vi "Joystick.vi"(8 "error in":errorcluster, 10 "error in Linx":errorcluster, 11 "LINX Ref":T1) -> (0 "error out":errorcluster, 1 "Signals":cluster{"Switch":bool, "Ultrasonic":dbl}, 2 "Joystick":T7, 3 "Refnum out":refnum<k1>, 4 "error out Linx":errorcluster, 5 "LINX Ref":T1)   [LabVIEW 2013]
uses:
  <vilib>/LabVIEW Hacker/LINX/Private/Type Defs/LINX Ref.ctl
  <vilib>/LabVIEW Hacker/LINX/Private/Type Defs/Platform.ctl
  <vilib>/LabVIEW Hacker/LINX/Private/Type Defs/Interface.ctl
  <vilib>/LabVIEW Hacker/LINX/Private/Device/Type Defs/LINX Device Config.ctl
  <vilib>/LabVIEW Hacker/LINX/Private/Device/Type Defs/TCP Config.ctl
  <vilib>/LabVIEW Hacker/LINX/Private/Type Defs/Device Family.ctl
  <vilib>/Utility/inputDevices.llb/joystickAcquire.vi
  <vilib>/LabVIEW Hacker/LINX/Public/Peripherals/Analog/Analog Read 1 Chan.vi
  <vilib>/LabVIEW Hacker/LINX/Public/Peripherals/Digital/Digital Read 1 Chan.vi
  <vilib>/LabVIEW Hacker/LINX/LVH-LINX.lvlib
  <vilib>/LabVIEW Hacker/LINX/Private/Device/Device.lvlib
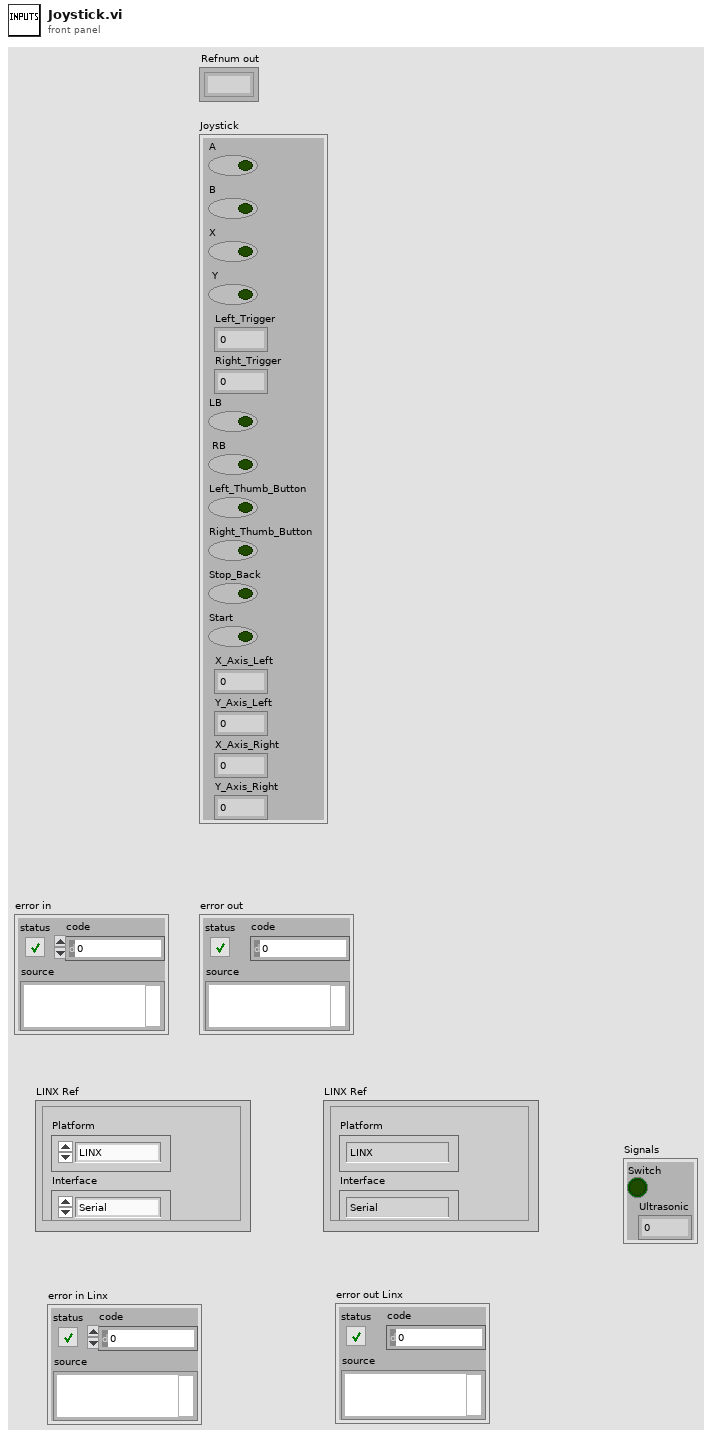
[diagram p1: front panel]
types:
  T1 = typedef "LVH-LINX.lvlib/LINX Ref.ctl" = cluster{"Platform":T2, "Interface":T3, "LINX Device Config":T4}
  T2 = typedef "LVH-LINX.lvlib/Platform.ctl" = enum16{"LINX", "myRIO"}
  T3 = typedef "LVH-LINX.lvlib/Interface.ctl" = enum16{"Serial", "TCP"}
  T4 = typedef "LVH-LINX.lvlib/Device.lvlib/LINX Device Config.ctl" = cluster{"Interface":T3, "COM Port":refnum<visa-resource-name>, "TCP Configuration":T5, "Device Family":T6, "Device ID":u8, "Device Name":string, "TCP Ref":refnum<k5>}
  T5 = typedef "LVH-LINX.lvlib/Device.lvlib/TCP Config.ctl" = cluster{"IP Address":string, "Port":u16}
  T6 = typedef "LVH-LINX.lvlib/Device Family.ctl" = enum8{"National Instruments", "Digilent", "Arduino"}
  T7 = cluster{"A":bool, "B":bool, "X":bool, " Y":bool, "Left_Trigger":dbl, "Right_Trigger ":dbl, "LB":bool, " RB":bool, "Left_Thumb_Button":bool, "Right_Thumb_Button":bool, "Stop_Back":bool, "Start":bool, "X_Axis_Left":dbl, "Y_Axis_Left":dbl, "X_Axis_Right":dbl, "Y_Axis_Right":dbl}
  T8 = cluster{"X axis":i32, "Y axis":i32, "Z axis":i32, "X axis rotation":i32, "Y axis rotation":i32, "Z axis rotation":i32, "U axis":i32, "V axis":i32}
  T9 = cluster{"button 1":bool, "button 2":bool, "button 3":bool, "button 4":bool, "button 5":bool, "button 6":bool, "button 7":bool, "button 8":bool, "button 9":bool, "button 10":bool, "button 11":bool, "button 12":bool, "button 13":bool, "button 14":bool, "button 15":bool, "button 16":bool, "button 17":bool, "button 18":bool, "button 19":bool, "button 20":bool, "button 21":bool, "button 22":bool, "button 23":bool, "button 24":bool, "button 25":bool, "button 26":bool, "button 27":bool, "button 28":bool, "button 29":bool, "button 30":bool, "button 31":bool, "button 32":bool}
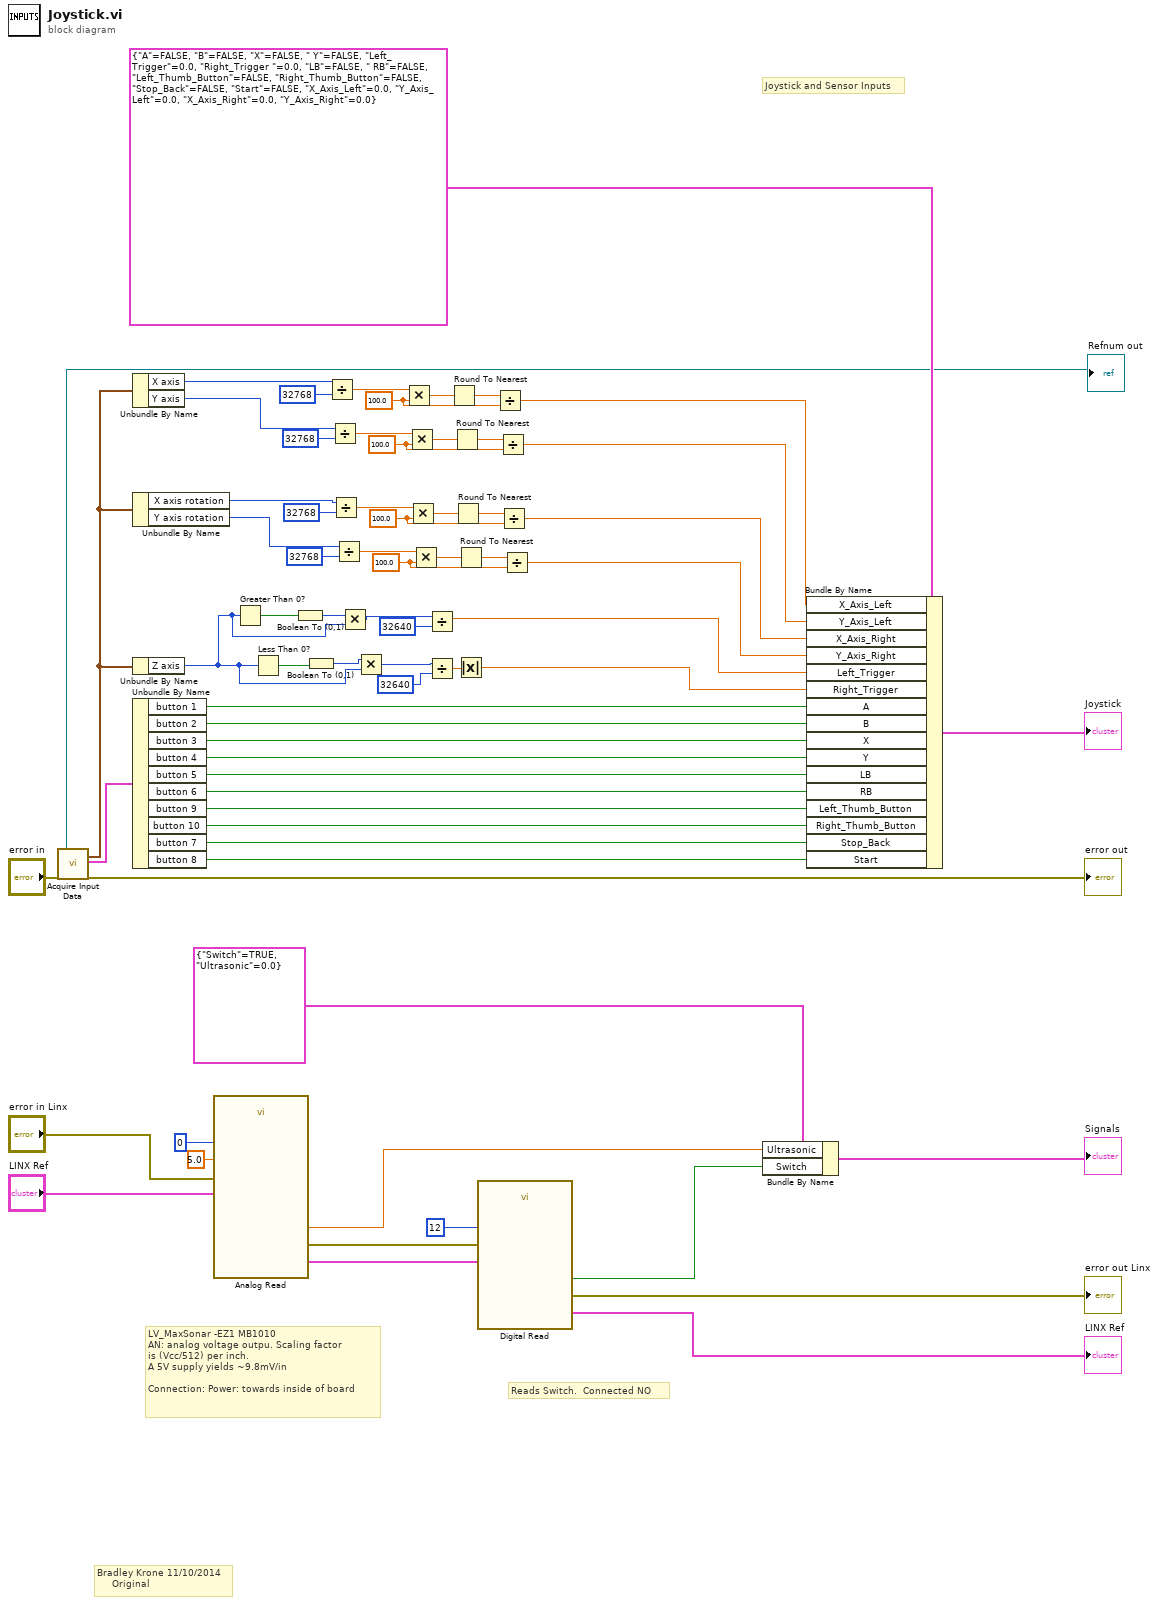
[diagram p0: block diagram]
diagram:
  w63 = 100.0 ("y")
  w58 = 100.0 ("y")
  w52 = 100.0 ("y")
  w47 = 100.0 ("y")
  # "Bradley Krone 11/10/2014\n     Original"
  # "Joystick and Sensor Inputs"
  # "Reads Switch.  Connected NO"
  # "LV_MaxSonar -EZ1 MB1010\nAN: analog voltage outpu. Scaling factor \nis (Vcc/512) per inch.  \nA 5V supply yields ~9.8mV/in\n\nConnection: Power: towards inside of board"
  n1 = call-poly <vilib>:"Acquire Input Data.vi"("error in (no error)"="error in") -> ("device ID"=→"Refnum out":refnum<k1>, "axis info"=w41:T8, "button info"=w16:T9, "error out"=→"error out":errorcluster)  [unwired: 1 in, 14 out]
  n2 = Unbundle By Name(w41) -> ("X axis"=w42:i32, "Y axis"=w53:i32)
  n3 = Unbundle By Name(w41) -> ("X axis rotation"=w64:i32, "Y axis rotation"=w65:i32)
  n4 = Unbundle By Name(w41) -> ("Z axis"=w37:i32)
  n5 = Unbundle By Name(w16) -> ("button 1"=w18:bool, "button 2"=w19:bool, "button 3"=w20:bool, "button 4"=w21:bool, "button 5"=w22:bool, "button 6"=w23:bool, "button 9"=w24:bool, "button 10"=w25:bool, "button 7"=w26:bool, "button 8"=w27:bool)
  n6 = call-poly <vilib>:"Analog Read.vi"("Analog Ref Override"=5.0, "Error In"="error in Linx", "Analog Channel"=0, "LINX Resource"="LINX Ref") -> ("Error Out"=w9:errorcluster, "AI Value"=w1:dbl, "LINX Resource"=w8:T1)  [unwired: 4 in, 1 out]
  n7 = Greater Than 0?(x=w37) -> (x > 0?=w30:bool)
  n8 = Less Than 0?(x=w37) -> (x < 0?=w35:bool)
  n9 = Boolean To (0,1)(Boolean=w30) -> (0, 1=w29:i16)
  n10 = Boolean To (0,1)(Boolean=w35) -> (0, 1=w36:i16)
  n11 = Divide(x=w42, y=32768) -> (x/y=w44:dbl)
  n12 = Divide(x=w53, y=32768) -> (x/y=w49:dbl)
  n13 = Divide(x=w64, y=32768) -> (x/y=w55:dbl)
  n14 = Divide(x=w65, y=32768) -> (x/y=w60:dbl)
  n15 = Multiply(x=w29, y=w37) -> (x*y=w32:i32)
  n16 = Multiply(x=w36, y=w37) -> (x*y=w38:i32)
  n17 = Multiply(x=w44, y=w47) -> (x*y=w45:dbl)
  n18 = Multiply(x=w49, y=w52) -> (x*y=w50:dbl)
  n19 = Multiply(x=w55, y=w58) -> (x*y=w56:dbl)
  n20 = Multiply(x=w60, y=w63) -> (x*y=w61:dbl)
  n21 = Divide(x=w32, y=32640) -> (x/y=w31:dbl)
  n22 = Divide(x=w38, y=32640) -> (x/y=w39:dbl)
  n23 = Round To Nearest(number=w45) -> (nearest integer value=w46:dbl)
  n24 = Round To Nearest(number=w50) -> (nearest integer value=w51:dbl)
  n25 = Round To Nearest(number=w56) -> (nearest integer value=w57:dbl)
  n26 = Round To Nearest(number=w61) -> (nearest integer value=w62:dbl)
  n27 = Absolute Value(x=w39) -> (abs(x)=w40:dbl)
  n28 = call-poly <vilib>:"Digital Read.vi"("Error In"=w9, "DI Channel"=12, "LINX Resource"=w8) -> ("Error Out"=→"error out Linx":errorcluster, "DI Value"=w3:bool, "LINX Resource"=→"LINX Ref":T1)  [unwired: 6 in]
  n29 = Divide(x=w46, y=w47) -> (x/y=w66:dbl)
  n30 = Divide(x=w51, y=w52) -> (x/y=w67:dbl)
  n31 = Divide(x=w57, y=w58) -> (x/y=w68:dbl)
  n32 = Divide(x=w62, y=w63) -> (x/y=w69:dbl)
  n33 = Bundle By Name(cluster=cluster{"Switch":bool, "Ultrasonic":dbl} {"Switch"=TRUE, "Ultrasonic"=0.0} ("Cluster"), "Ultrasonic"=w1, "Switch"=w3) -> (→"Signals":cluster{"Switch":bool, "Ultrasonic":dbl})
  n34 = Bundle By Name(cluster=T7 {"A"=FALSE, "B"=FALSE, "X"=FALSE, " Y"=FALSE, "Left_Trigger"=0.0, "Right_Trigger "=0.0, "LB"=FALSE, " RB"=FALSE, "Left_Thumb_Button"=FALSE, "Right_Thumb_Button"=FALSE, "Stop_Back"=FALSE, "Start"=FALSE, "X_Axis_Left"=0.0, "Y_Axis_Left"=0.0, "X_Axis_Right"=0.0, "Y_Axis_Right"=0.0}, "X_Axis_Left"=w66, "Y_Axis_Left"=w67, "X_Axis_Right"=w68, "Y_Axis_Right"=w69, "Left_Trigger"=w31, "Right_Trigger"=w40, "A"=w18, "B"=w19, "X"=w20, "Y"=w21, "LB"=w22, "RB"=w23, "Left_Thumb_Button"=w24, "Right_Thumb_Button"=w25, "Stop_Back"=w26, "Start"=w27) -> (→"Joystick":T7)
